vi "Tom Filter.vi"(10 "Tom":bool, 11 "Data In":waveform(dbl)[](array[waveform])) -> (3 "Data out":waveform(dbl)[](array[waveform]))   [LabVIEW 2022 SP3]
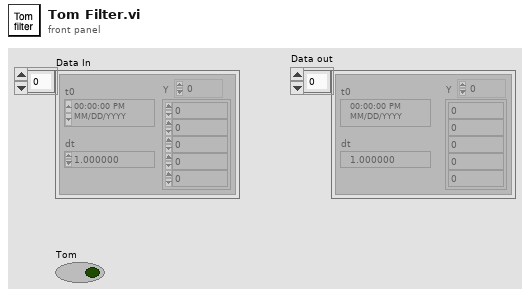
[diagram p1: front panel]
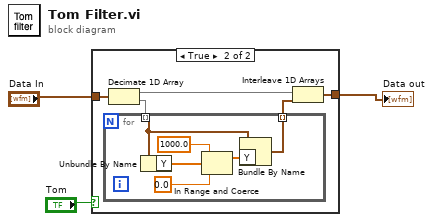
[diagram p0: block diagram]
diagram:
  n1 = case shown="True" "Tom" {
    tunnel: "Data In" -> [w4 w9]
    tunnel: [w4 w7] -> w3
    frame False {
    }
    frame True {
      n2 = Decimate 1D Array(w9) -> (w8:waveform(dbl)[], w6:waveform(dbl)[])
      n3 = for {
        tunnel: [w14] -> w5 mode=indexing
        tunnel: w6 -> [w15] mode=indexing
        n4 = Unbundle By Name(w15) -> ("Y"=w13:dbl[])
        n5 = In Range and Coerce(upper limit=1000.0, x=w13, lower limit=0.0) -> (coerced(x)=w12:dbl[])  [unwired: 1 out]
        n6 = Bundle By Name(cluster=w15, "Y"=w12) -> (w14:waveform(dbl))
      }
      n7 = Interleave 1D Arrays(w8, w5) -> (w7:waveform(dbl)[])
    }
  }
  "Data out" <- w3
